vi "CRYUpdate Tree for Load.vi"(8 "Is Move?":bool, 10 "ProjectViewCluster In":T1, 11 "RefTree In":refnum<vi>) -> (3 "RefTree Out":refnum<vi>)   [LabVIEW 2013]
uses:
  CRYSystem/Typedef Control/CRYProjectViewCluster.ctl
  CRYProject Editor Global.vi
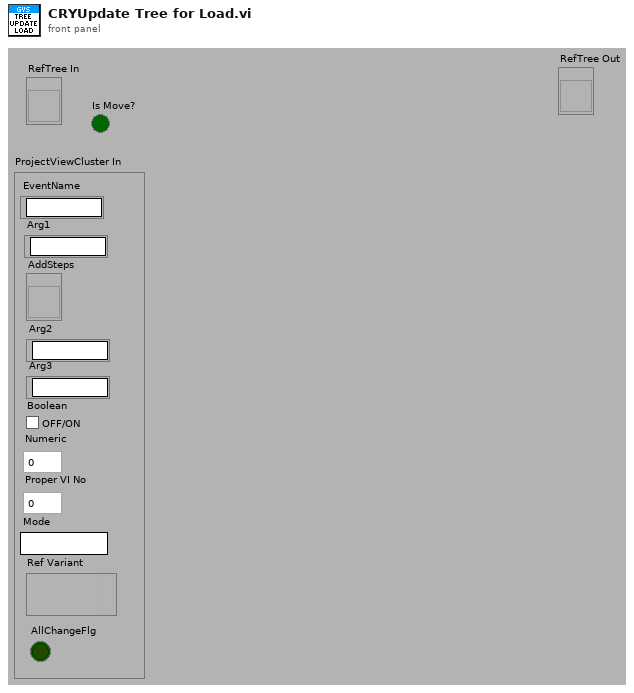
[diagram p1: front panel]
types:
  T1 = typedef "CRYProjectViewCluster.ctl" = cluster{"EventName":string, "Arg1":string, "Numeric":i32, "Proper VI No":i32, "AddSteps ":refnum<vi>, "Arg2":string, "Arg3":string, "Boolean":bool, "Mode":string, "Ref Variant":variant, "AllChangeFlg":bool}
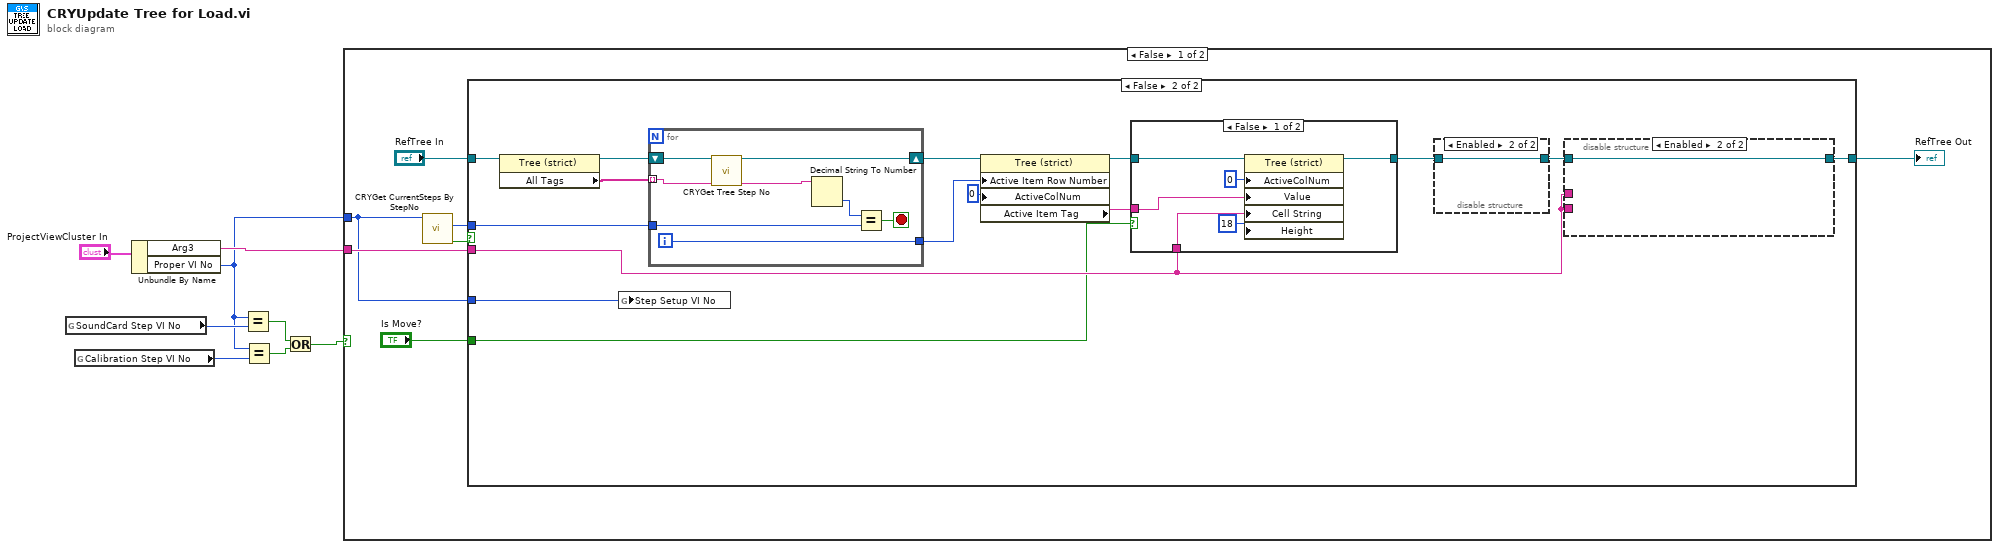
[diagram p0: block diagram]
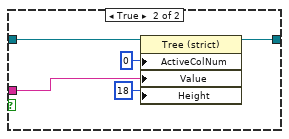
[diagram p3: hidden frame]
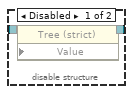
[diagram p4: hidden frame]
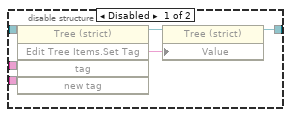
[diagram p5: hidden frame]
diagram:
  n1 = global read "CRYProject Editor Global.vi" "SoundCard Step VI No"() -> (w6:i32)
  n2 = global read "CRYProject Editor Global.vi" "Calibration Step VI No"() -> (w4:i32)
  n3 = Unbundle By Name("ProjectViewCluster In") -> ("Arg3"=w7:string, "Proper VI No"=w5:i32)
  n4 = Equal?(x=w5, y=w6) -> (x = y?=w3:bool)
  n5 = Equal?(x=w5, y=w4) -> (x = y?=w2:bool)
  n6 = Or(x=w3, y=w2) -> (x .or. y?=w1:bool)
  n7 = case shown="False" w1 {
    tunnel: w7 -> [w13 _]
    tunnel: w5 -> [w9 _]
    frame False {
      n8 = call "CRYGet CurrentSteps By StepNo.vi"("Step Setup VI No"=w9) -> ("bResult"=w10:bool, "Index"=w11:i32)  [unwired: 8 in, 1 out]
      n9 = case shown="False" w10 {
        tunnel: [w16 w31] -> w15
        tunnel: w9 -> [_ w30]
        tunnel: "RefTree In" -> [w16 w26]
        tunnel: w13 -> [_ w19]
        tunnel: "Is Move?" -> [_ w18]
        tunnel: w11 -> [_ w17]
        frame True {
        }
        frame False {
          n10 = property on="Property Node" class="Tree (strict)"(reference=w26) -> (reference out=w29:refnum<vi>, "All Tags"=w28:string[])  [unwired: 1 in, 1 out]
          n11 = global write "CRYProject Editor Global.vi" "Step Setup VI No"(w30) -> ()
          n12 = for {
            tunnel: w28 -> [w48] mode=indexing
            tunnel: w17 -> [w52]
            tunnel: [w50] -> w24
            shift-right: [w46] -> w27
            shift-left: w29 -> [w49]
            i -> [w50]
            stop <- w51 stop-if-true
            n13 = call "CRYGet Tree Step No.vi"("SequenceTree"=w49, "Active Item Tag"=w48) -> ("reference out"=w46:refnum<vi>, "Active Cell String4"=w47:string)  [unwired: 12 in]
            n14 = Decimal String To Number(string=w47) -> (number=w53:i32)  [unwired: 2 in, 1 out]
            n15 = Equal?(x=w53, y=w52) -> (x = y?=w51:bool)
          }
          n16 = property on="Property Node" class="Tree (strict)"(reference=w27, "Active Item Row Number"=w24, "ActiveColNum"=0 ("Active Cell:Active Column Number")) -> (reference out=w25:refnum<vi>, "Active Item Tag"=w20:string)  [unwired: 1 in, 1 out]
          n17 = case shown="False" w18 {
            tunnel: w25 -> [w37 w41]
            tunnel: [w36 w40] -> w23
            tunnel: w20 -> [w34 w39]
            tunnel: w19 -> [w33 _]
            frame False {
              n18 = property on="Property Node" class="Tree (strict)"(reference=w37, "ActiveColNum"=0 ("Active Cell:Active Column Number"), "Value"=w34, "Cell String"=w33, "Height"=18 ("Active Cell:Cell Size:Height")) -> (reference out=w36:refnum<vi>)  [unwired: 1 in, 1 out]
            }
            frame True {
              n19 = property on="Property Node" class="Tree (strict)"(reference=w41, "ActiveColNum"=0 ("Active Cell:Active Column Number"), "Value"=w39, "Height"=18 ("Active Cell:Cell Size:Height")) -> (reference out=w40:refnum<vi>)  [unwired: 1 in, 1 out]
            }
          }
          n20 = disable-structure shown="Enabled" {
            disable-tunnel: w23 -> [w44 w45]
            disable-tunnel: [w43 w45] -> w22
            frame Disabled {
              n21 = property on="Property Node" class="Tree (strict)" props=["Value"](reference=w44) -> (reference out=w43:refnum<vi>)  [unwired: 2 in, 1 out]
            }
            frame Enabled {
            }
          }
          n22 = disable-structure shown="Enabled" {
            disable-tunnel: [w58 w60] -> w31
            disable-tunnel: w19 -> [w57 _]
            disable-tunnel: w22 -> [w56 w60]
            disable-tunnel: w19 -> [w54 _]
            frame Disabled {
              n23 = invoke class="Tree (strict)" method="Edit Tree Items.Set Tag"(reference=w56, "tag"=w57, "new tag"=w54) -> (reference out=w55:refnum<vi>, "Edit Tree Items:Set Tag"=w59:string)  [unwired: 2 in, 3 out]
              n24 = property on="Property Node" class="Tree (strict)"(reference=w55, "Value"=w59) -> (reference out=w58:refnum<vi>)  [unwired: 1 in, 1 out]
            }
            frame Enabled {
            }
          }
        }
      }
      "RefTree Out" <- w15
    }
    frame True {
    }
  }
